vi "ACCELL_TEST.vi"() -> ()   [LabVIEW 2010]
uses:
  <vilib>/NXT/Block Support/NXT_InputPort.ctl
  subVIs/dIMU_Accel_gs.vi
panel:
  out "Z Accel (g)":dbl
  out "Y Accel (g)":dbl
  out "X Accel (g)":dbl
  in  "Boolean":bool
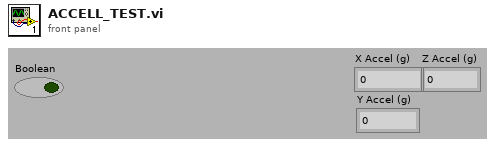
[diagram p1: front panel]
types:
  T1 = typedef "NXT_InputPort.ctl" = u8
  T2 = typedef "LVHSConnector.ctl" = cluster{"Hardware":string, "Flattened String":string}
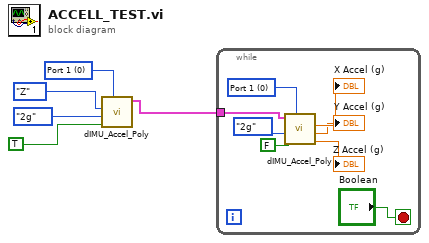
[diagram p0: block diagram]
diagram:
  w3 = T1 0 items=["Port 1", "Port 2", "Port 3", "Port 4"] ("Port")
  n1 = call-poly "dIMU_Accel_Poly.vi"("Port"=w3, "Calibrate"=TRUE, "Maximum Range"=enum8{"2g", "4g", "8g"}."2g", "Calibrate Axis"=enum8{"Z", "X", "Y"}."Z") -> ("NXT"=w2:T2)  [unwired: 4 in, 3 out]
  n2 = while {
    tunnel: w2 -> [w9]
    stop <- "Boolean" stop-if-true
    w10 = T1 0 items=["Port 1", "Port 2", "Port 3", "Port 4"] ("Port")
    n3 = call-poly "dIMU_Accel_Poly.vi"("Port"=w10, "Calibrate"=FALSE, "Maximum Range"=enum8{"2g", "4g", "8g"}."2g", "NXT"=w9) -> ("Z Accel (g)"=→"Z Accel (g)":dbl, "Y Accel (g)"=→"Y Accel (g)":dbl, "X Accel (g)"=→"X Accel (g)":dbl)  [unwired: 4 in, 1 out]
  }
